vi "lockin - add phase element.vi"(8 "error in (no error)":errorcluster, 11 "LockinDAQ":refnum<class "LockinDAQ.lvclass">) -> (0 "error out":errorcluster, 3 "LockinDAQ out":refnum<class "LockinDAQ.lvclass">)   [LabVIEW 2016, in "LockinDAQ.lvclass"]
uses:
  LockinDAQ.lvclass
  LockinDAQ.lvclass/LockinDAQ.ctl
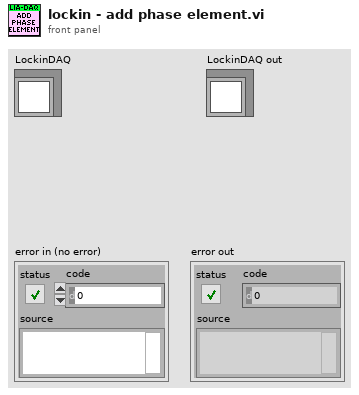
[diagram p1: front panel]
types:
  T1 = typedef "LockinDAQ.lvclass/REF-cluster.ctl" = cluster{"REF f (Hz)":T2, "REF phi (°)":T3}
  T2 = typedef "LockinDAQ.lvclass/REF_f-array.ctl" = dbl[]
  T3 = typedef "LockinDAQ.lvclass/REF_phi-array.ctl" = dbl[]
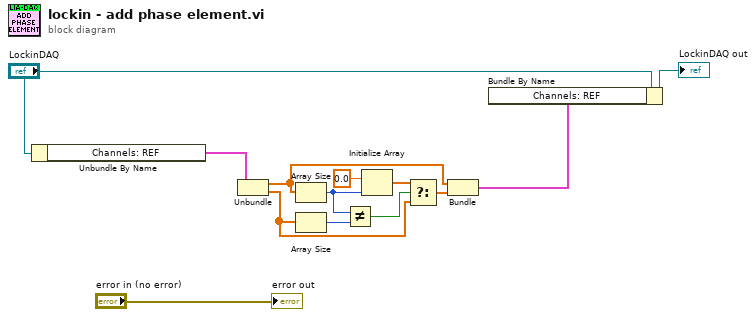
[diagram p0: block diagram]
diagram:
  n1 = Unbundle By Name("LockinDAQ") -> ("Channels: REF"=w5:T1)
  n2 = Unbundle(w5) -> ("REF f (Hz)"=w11:T2, "REF phi (°)"=w9:T3)
  n3 = Array Size(array=w11) -> (size(s)=w6:i32)
  n4 = Array Size(array=w9) -> (size(s)=w12:i32)
  n5 = Not Equal?(x=w6, y=w12) -> (x != y?=w13:bool)
  n6 = Initialize Array(0.0 ("element"), w6) -> (w8:dbl[])
  n7 = Select(t=w8, s=w13, f=w9) -> (s? t:f=w10:T3)
  n8 = Bundle("REF f (Hz)"=w11, "REF phi (°)"=w10) -> (w2:cluster{"REF f (Hz)":T2, "REF phi (°)":T3})  [unwired: 1 in]
  n9 = Bundle By Name(cluster="LockinDAQ", "Channels: REF"=w2) -> (→"LockinDAQ out":refnum<class "LockinDAQ.lvclass">)
  "error out" <- "error in (no error)"
